vi "Stop Action.vi"(8 "error in (no error)":errorcluster, 11 "Device in":refnum<class "Device.lvclass">) -> (0 "error out":errorcluster, 3 "Device out":refnum<class "Device.lvclass">)   [LabVIEW 2023, in "Device.lvlib" / "Device.lvclass"]
uses:
  Device.lvclass
  Device.lvclass/Device.ctl
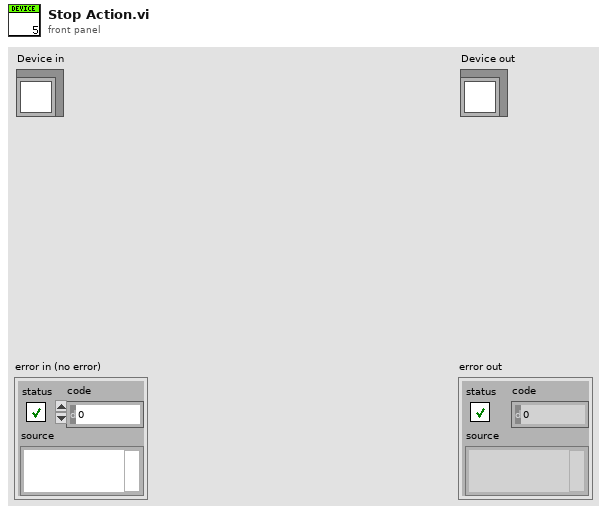
[diagram p1: front panel]
types:
  T1 = typedef "Device.lvlib/Device.lvclass/cyclical pattern.ctl" = enum16{"No Loop", "Fastest", "Timer"}
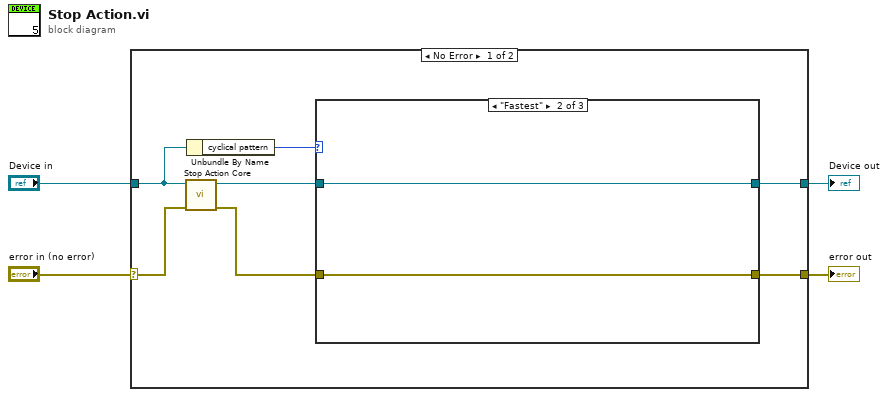
[diagram p0: block diagram]
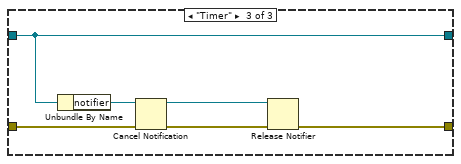
[diagram p3: hidden frame]
diagram:
  n1 = case shown="No Error" "error in (no error)" {
    selector: "error in (no error)" -> [w11 w23]
    tunnel: [w6 w23] -> w3
    tunnel: [w5 w22] -> w1
    tunnel: "Device in" -> [w10 w22]
    frame No Error {
      n2 = call-dynamic "Stop Action Core.vi"("error in (no error)"=w11, "Device in"=w10) -> ("error out"=w7:errorcluster, "Device out"=w9:refnum<class "Device.lvclass">)  [unwired: 8 in]
      n3 = Unbundle By Name(w10) -> ("cyclical pattern"=w8:T1)
      n4 = case shown="\"Fastest\"" w8 {
        tunnel: w9 -> [w12 w14 w19]
        tunnel: w7 -> [w13 w15 w21]
        tunnel: [w13 w15 w16] -> w6
        tunnel: [w12 w14 w19] -> w5
        frame "No Loop", Default {
        }
        frame "Fastest" {
        }
        frame "Timer" {
          n5 = Unbundle By Name(w19) -> ("notifier"=w20:refnum<notifier>)
          n6 = Cancel Notification(0:w20, 3:w21) -> (8:w17:refnum<notifier>, 11:w18:errorcluster)  [unwired: 1 out]
          n7 = Release Notifier(notifier=w17, error in (no error)=w18) -> (error out=w16:errorcluster)  [unwired: 1 in, 2 out]
        }
      }
    }
    frame Error {
    }
  }
  "error out" <- w3
  "Device out" <- w1
